vi "Set Control AttributeValue.vi"(8 "error in (no error)":errorcluster, 10 "AttributeValue":variant, 11 "UIConfiguration in":refnum<class "UIConfiguration.lvclass">) -> (0 "error out":errorcluster, 3 "UIConfiguration out":refnum<class "UIConfiguration.lvclass">)   [LabVIEW 2015, in "UIConfiguration.lvclass"]
uses:
  UIConfiguration.lvclass
  UIConfiguration.lvclass/UIConfiguration.ctl
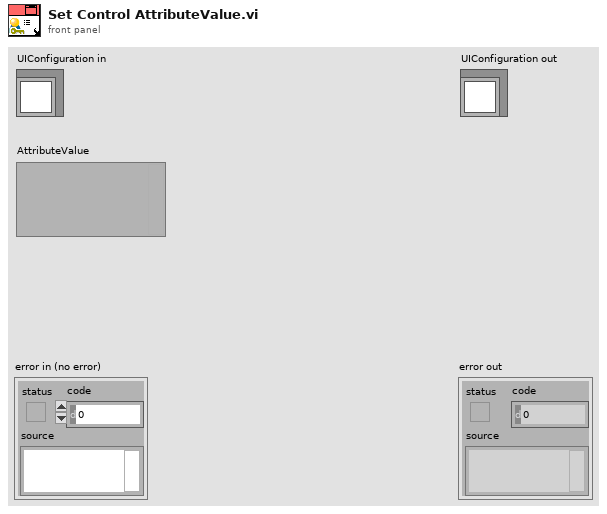
[diagram p1: front panel]
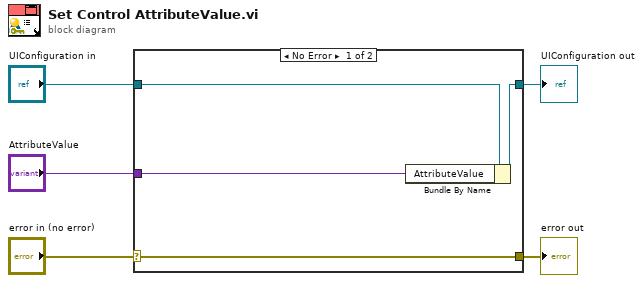
[diagram p0: block diagram]
diagram:
  n1 = case shown="No Error" "error in (no error)" {
    selector: "error in (no error)" -> [w9 w10]
    tunnel: [w9 w10] -> w4
    tunnel: [w7 w11] -> w2
    tunnel: "UIConfiguration in" -> [w8 w11]
    tunnel: "AttributeValue" -> [w6 _]
    frame No Error {
      n2 = Bundle By Name(cluster=w8, "AttributeValue"=w6) -> (w7:refnum<class "UIConfiguration.lvclass">)
    }
    frame Error {
    }
  }
  "error out" <- w4
  "UIConfiguration out" <- w2
